vi "Write Element Writer.vi"(10 "Abstract Param Writer.lvclass":refnum<class "Abstract Param Writer.lvclass">, 11 "Array Writer in":refnum<class "Array Writer.lvclass">) -> (3 "Array Writer out":refnum<class "Array Writer.lvclass">)   [LabVIEW 2013, in "Array Writer.lvclass"]
doc: "Copyright (c) 2016 Sze Howe Koh\n\nThis Source Code Form is subject to the terms of the Mozilla Public License, v. 2.0. If a copy of the MPL was not distributed with this file, You can obtain one at http://mozilla.org/MPL/2.0/."
uses:
  Array Writer.lvclass
  Abstract Param Writer/Abstract Param Writer.lvclass
  Array Writer.lvclass/Array Writer.ctl
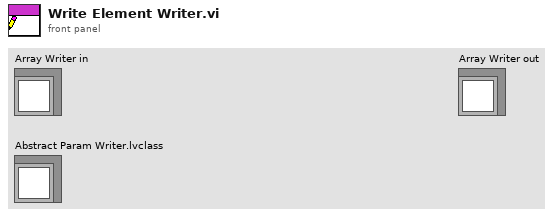
[diagram p1: front panel]
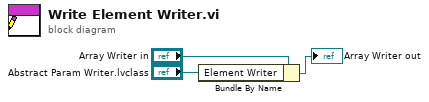
[diagram p0: block diagram]
diagram:
  n1 = Bundle By Name(cluster="Array Writer in", "Element Writer"="Abstract Param Writer.lvclass") -> (→"Array Writer out":refnum<class "Array Writer.lvclass">)
